vi "Handle INSERT Error.vi"(8 "error in (no error)":errorcluster, 10 "SQL":string, 11 "Database.PG":refnum<class "Data.PGSQL.lvclass">) -> (0 "error out":errorcluster, 2 "Wrote to DB?":bool, 3 "Database.PG out":refnum<class "Data.PGSQL.lvclass">)   [LabVIEW 2013, in "Data.PGSQL.lvclass"]
uses:
  Data.PGSQL.lvclass
  <vilib>/Utility/sysdir.llb/System Directory Type.ctl
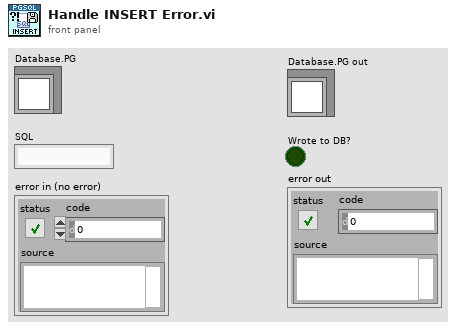
[diagram p1: front panel]
types:
  T1 = typedef "System Directory Type.ctl" = i32
  T2 = enum16{"open", "replace", "create", "open or create", "replace or create", "replace or create with confirmation"}
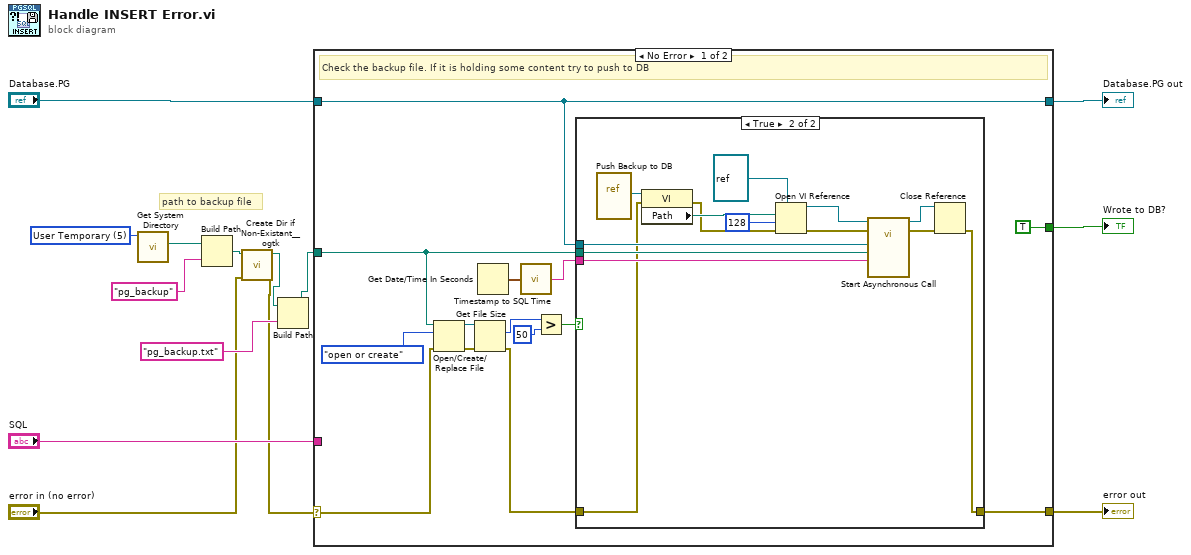
[diagram p0: block diagram]
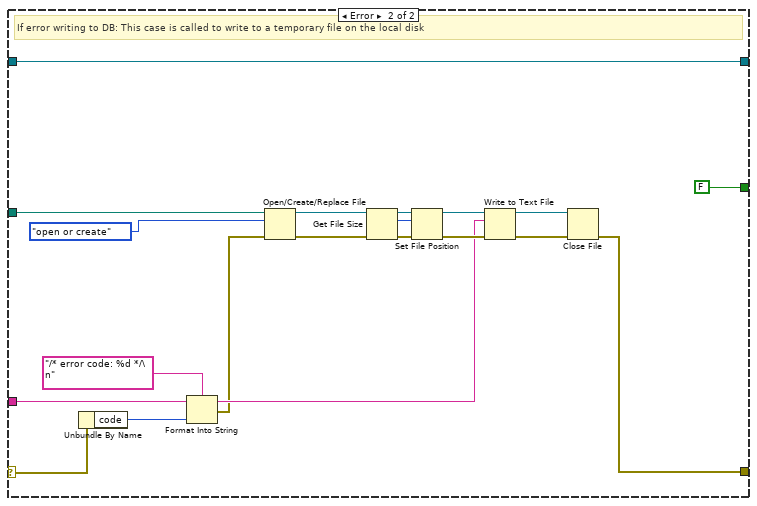
[diagram p3: hidden frame]
diagram:
  w14 = T1 5 items=["User Home"=0, "User Desktop"=1, "User Documents"=2, "User Application Data"=3, "User Preferences"=4, "User Temporary"=5, "Public Documents"=6, "Public Application Data"=7, "Public Preferences"=8, "Public Cache"=13, "System Core Libraries"=9, "System Installed Libraries"=10, "Application Files"=11, "Boot Volume Root"=12] ("system directory type")
  # "path to backup file"
  n1 = call <vilib>:"Get System Directory.vi"("system directory type"=w14) -> ("system directory"=w13:path)  [unwired: 10 in]
  n2 = Build Path(base path=w13, name or relative path="pg_backup") -> (appended path=w6:path)
  n3 = call "Create Dir if Non-Existant__ogtk.vi"("error in (no error)"="error in (no error)", "Directory Path"=w6) -> ("error out"=w1:errorcluster, "dup Directory Path"=w5:path)  [unwired: 7 in, 1 out]
  n4 = Build Path(base path=w5, name or relative path="pg_backup.txt") -> (appended path=w4:path)
  n5 = case shown="No Error" w1 {
    selector: w1 -> [w18 w45]
    tunnel: "SQL" -> [_ w63]
    tunnel: [TRUE FALSE] -> w9
    tunnel: "Database.PG" -> [w17 w48]
    tunnel: w4 -> [w16 w49]
    tunnel: [w17 w48] -> w8
    tunnel: [w19 w46] -> w7
    frame No Error {
      # "Check the backup file. If it is holding some content try to push to DB"
      n6 = Open/Create/Replace File(file path (use dialog)=w16, error in=w18, operation (0:open)=T2."open or create") -> (refnum out=w27:refnum<file>, error out=w28:errorcluster)  [unwired: 3 in, 1 out]
      n7 = Get File Size(file=w27, error in=w28) -> (size (in bytes)=w26:i64, 0:w15:errorcluster)  [unwired: 1 out]
      n8 = Get Date/Time In Seconds() -> (seconds since 1Jan1904=w21:timestamp)
      n9 = call "Timestamp to SQL Time.vi"("seconds since 1Jan1904"=w21) -> ("date/time string"=w20:string)
      n10 = Greater?(x=w26, y=i64 50) -> (0:w23:bool)
      n11 = case shown="True" w23 {
        tunnel: w20 -> [_ w41]
        tunnel: w17 -> [_ w35]
        tunnel: w16 -> [_ w42]
        tunnel: [w29 w34] -> w19
        tunnel: w15 -> [w29 w30]
        frame False {
        }
        frame True {
          n12 = vi-ref "Push Backup to DB.vi"() -> (w33:refnum<vi>)
          n13 = property class="VI"(reference=w33, error in=w30) -> (error out=w31:errorcluster, "Path"=w32:path)  [unwired: 1 out]
          n14 = Open VI Reference(type specifier VI Refnum (for type only)=refnum<vi> refnum, vi path=w32, options=128, error in (no error)=w31) -> (vi reference=w40:refnum<vi>, error out=w38:errorcluster)  [unwired: 2 in]
          n15 = call-by-ref "Start Asynchronous Call"(reference=w40, error in=w38, "timestamp string"=w41, "Path to backup file"=w42, "Data.PG in"=w35) -> (reference out=w36:refnum<vi>, error out=w39:errorcluster)  [unwired: 9 in]
          n16 = Close Reference(reference=w36, error in (no error)=w39) -> (error out=w34:errorcluster)
        }
      }
    }
    frame Error {
      # "If error writing to DB: This case is called to write to a temporary file on the local disk"
      n17 = Unbundle By Name(w45) -> ("code"=w50:i32)
      n18 = Format Into String(format string="/* error code: %d */\n", initial string=w63, w50) -> (resulting string=w57:string, error out=w47:errorcluster)  [unwired: 1 in]
      n19 = Open/Create/Replace File(file path (use dialog)=w49, error in=w47, operation (0:open)=T2."open or create") -> (refnum out=w53:refnum<file>, error out=w52:errorcluster)  [unwired: 3 in, 1 out]
      n20 = Get File Size(file=w53, error in=w52) -> (refnum out=w60:refnum<file>, size (in bytes)=w61:i64, 0:w62:errorcluster)
      n21 = Set File Position(offset (in bytes) (0)=w61, refnum=w60, error in=w62) -> (refnum out=w58:refnum<file>, error out=w59:errorcluster)  [unwired: 1 in]
      n22 = Write to Text File(file (use dialog)=w58, text=w57, error in=w59) -> (refnum out=w55:refnum<file>, error out=w56:errorcluster)  [unwired: 1 in, 1 out]
      n23 = Close File(refnum=w55, error in=w56) -> (error out=w46:errorcluster)  [unwired: 1 out]
    }
  }
  "Wrote to DB?" <- w9
  "Database.PG out" <- w8
  "error out" <- w7
